vi "_PC_Pub_FM setSampleType.vi"(8 "error in (no error)":errorcluster, 11 "FM in":refnum<class "FM.lvclass">) -> (0 "error out":errorcluster, 3 "FM out":refnum<class "FM.lvclass">)   [LabVIEW 2018, in "FM.lvclass"]
uses:
  FM.lvclass
  FM.lvclass/FM.ctl
  DataXML/DataXML.lvclass
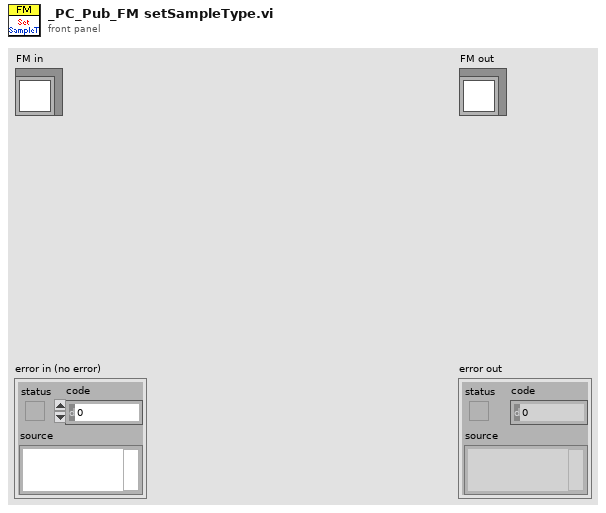
[diagram p1: front panel]
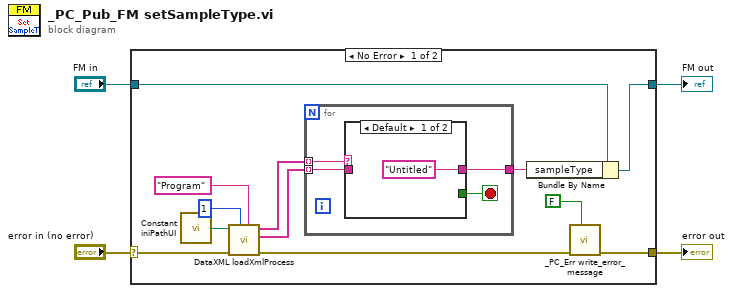
[diagram p0: block diagram]
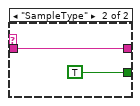
[diagram p2: hidden frame]
diagram:
  n1 = case shown="No Error" "error in (no error)" {
    selector: "error in (no error)" -> [w11 w25]
    tunnel: [w5 w25] -> w3
    tunnel: [w8 w24] -> w1
    tunnel: "FM in" -> [w10 w24]
    frame No Error {
      n2 = call "Constant iniPathUI.vi"() -> ("appended path"=w12:path)
      n3 = call "DataXML loadXmlProcess.vi"("target name"="Program", "level"=u8 1, "error in (no error)"=w11, "xml_data_path"=w12) -> ("error IO"=w6:errorcluster, "value"=w16:string[], "name"=w15:string[])  [unwired: 4 in, 1 out]
      n4 = for {
        tunnel: w15 -> [w20] mode=indexing
        tunnel: w16 -> [w19] mode=indexing
        tunnel: [w18] -> w9
        stop <- w17 stop-if-true
        n5 = case shown="Default" w20 {
          tunnel: w19 -> [_ w23]
          tunnel: ["Untitled" ("Value") w23] -> w18
          tunnel: [_ TRUE] -> w17
          frame Default {
          }
          frame "SampleType" {
          }
        }
      }
      n6 = Bundle By Name(cluster=w10, "sampleType"=w9) -> (w8:refnum<class "FM.lvclass">)
      n7 = call "_PC_Err write_error_message.vi"("show msg( T )"=FALSE, "error in"=w6) -> ("error out"=w5:errorcluster)  [unwired: 9 in]
    }
    frame Error {
    }
  }
  "error out" <- w3
  "FM out" <- w1
